vi "CreateDataFile.vi"(6 "y轴标尺号":i32[](array[numeric]), 8 "y轴名称":string[](array[string]), 9 "header":string, 10 "suffix":string, 11 "dir path":string) -> (0 "error out":errorcluster, 2 "file path":path, 3 "refnum out":refnum<file>)   [LabVIEW 2020]
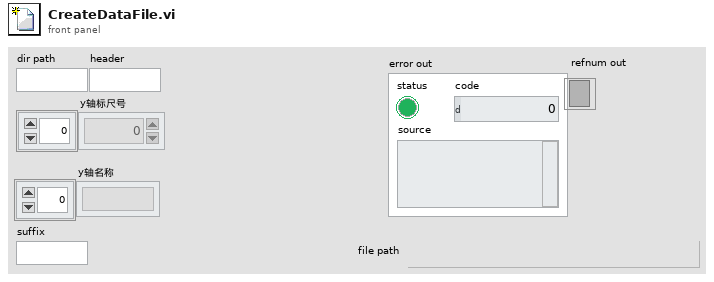
[diagram p1: front panel]
types:
  T1 = enum16{"open", "replace", "create", "open or create", "replace or create", "replace or create with confirmation"}
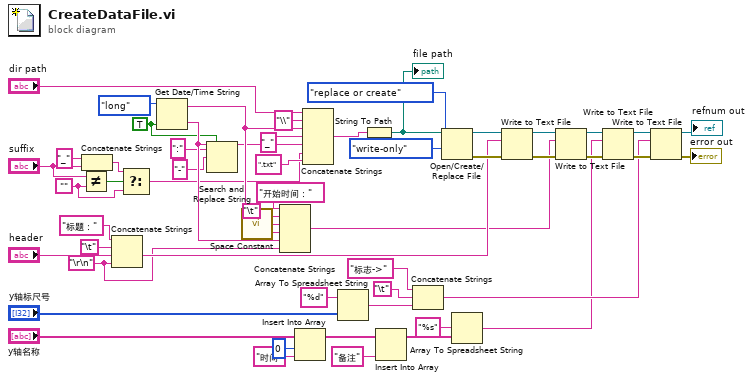
[diagram p0: block diagram]
diagram:
  w4 = "\r\n"
  w12 = ""
  w46 = TRUE ("需要秒？(F)")
  n1 = Not Equal?(x="suffix", y=w12) -> (x != y?=w13:bool)
  n2 = Concatenate Strings("_" ("string"), "suffix") -> (w10:string)
  n3 = Concatenate Strings("标题：" ("string"), "\t", "header", w4) -> (w8:string)
  n4 = Select(t=w10, s=w13, f=w12) -> (s? t:f=w11:string)
  n5 = Get Date/Time String(date format (0)=enum16{"short", "long", "abbreviated"}."long" ("日期格式(0)"), want seconds? (F)=w46) -> (date string=w48:string, time string=w49:string)  [unwired: 1 in]
  n6 = Search and Replace String(replace all?=w46, input string=w49, search string=":", replace string="-" ("replace string (\"\")")) -> (result string=w31:string)  [unwired: 4 in, 3 out]
  n7 = call <vilib>:"Space Constant.vi"() -> ("String"=w47:string)
  n8 = Concatenate Strings ("连接字符串")("开始时间：" ("字符串"), "\t", w48, w47, w49, w4) -> (w5:string)
  n9 = Insert Into Array(array="y轴名称", index=0 ("索引"), new element="时间" ("新元素/子数组")) -> (w42:string[])
  n10 = Concatenate Strings ("连接字符串")("dir path", "\\" ("字符串"), w48, "_" ("string"), w31, w11, ".txt" ("string")) -> (w52:string)
  n11 = Array To Spreadsheet String(array="y轴标尺号", 3:"%d" ("format string")) -> (spreadsheet string=w39:string)  [unwired: 1 in]
  n12 = String To Path(string=w52) -> (path=w51:path)
  "file path" <- w51
  n13 = Insert Into Array(array=w42, new element="备注" ("新元素/子数组")) -> (w43:string[])  [unwired: 1 in]
  n14 = Concatenate Strings("标志->" ("字符串"), "\t", w39) -> (w7:string)
  n15 = Open/Create/Replace File(file path (use dialog)=w51, operation (0:open)=T1."replace or create", access (0:read/write)=enum16{"read/write", "read-only", "write-only"}."write-only") -> (refnum out=w18:refnum<file>, error out=w17:errorcluster)  [unwired: 3 in, 1 out]
  n16 = Array To Spreadsheet String(array=w43, 3:"%s" ("format string")) -> (spreadsheet string=w6:string)  [unwired: 1 in]
  n17 = Write to Text File(file (use dialog)=w18, text=w8, error in=w17) -> (refnum out=w19:refnum<file>, error out=w20:errorcluster)  [unwired: 1 in, 1 out]
  n18 = Write to Text File(file (use dialog)=w19, text=w5, error in=w20) -> (refnum out=w37:refnum<file>, error out=w38:errorcluster)  [unwired: 1 in, 1 out]
  n19 = Write to Text File(file (use dialog)=w37, text=w6, error in=w38) -> (refnum out=w28:refnum<file>, error out=w27:errorcluster)  [unwired: 1 in, 1 out]
  n20 = Write to Text File(file (use dialog)=w28, text=w7, error in=w27) -> (refnum out=→"refnum out":refnum<file>, error out=→"error out":errorcluster)  [unwired: 1 in, 1 out]
